vi "PH_VacuumControl.prepare historical Multi Data.vi"(5 "Continue Fit":dbl, 6 "Pressure Data 1 [mbar]":dbl[](array[numeric]), 7 "Start Fit":dbl, 8 "Limit":dbl, 9 "Timebase [s]":i32[](array[numeric]), 10 "Pressure Data 2 [mbar]":dbl[](array[numeric])) -> (1 "Trend":cluster{i32[], "Data":dbl[]}[](graph), 2 "Time to reach Limit":dbl)   [LabVIEW 2014, in "PH_VacuumControl.lvlib"]
doc: "Within this VI the data are prepared for presentation at the GUI and a trend calculation is tried."
uses:
  PH_VacuumControl.lvlib
  <vilib>/Analysis/NI_AALPro.lvlib
panel:
  in  "parameter bounds":T1={"amp min"=-inf, "amp max"=inf, "damping min"=-inf, "damping max"=inf, "offset min"=0.0, "offset max"=0.0}
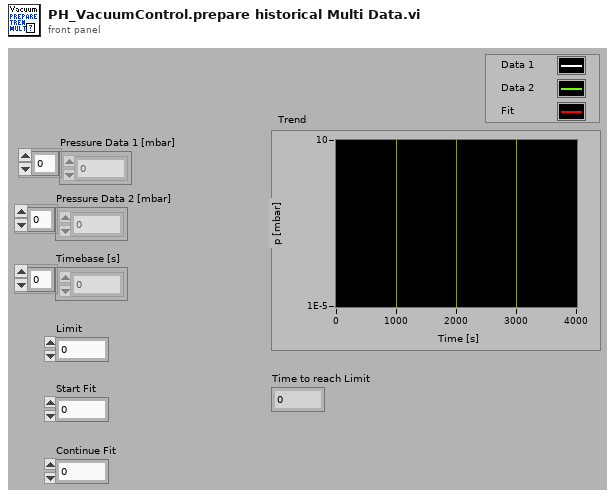
[diagram p1: front panel]
types:
  T1 = cluster{"amp min":dbl, "amp max":dbl, "damping min":dbl, "damping max":dbl, "offset min":dbl, "offset max":dbl}
  T2 = cluster{"Timebase [s]":i32[], "Pressure Data 1 [mbar]":dbl[]}
  T3 = cluster{"Timebase [s]":i32[], "Pressure Data 2 [mbar]":dbl[]}
  T4 = cluster{"Timebase [s]":i32[], "Best Exponential Fit":dbl[]}[]
  T5 = cluster{"Timebase [s]":i32[], "Pressure Data 2 [mbar]":dbl[]}[]
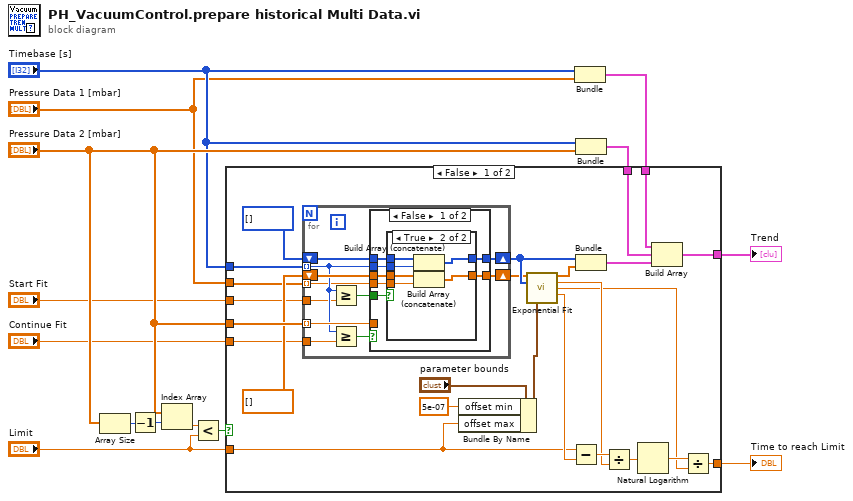
[diagram p0: block diagram]
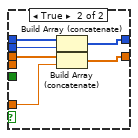
[diagram p3: hidden frame]
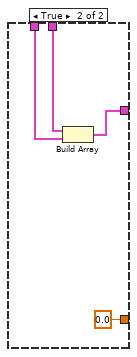
[diagram p4: hidden frame]
diagram:
  n1 = Array Size(array="Pressure Data 2 [mbar]") -> (size(s)=w13:i32)
  n2 = Decrement(x=w13) -> (x-1=w11:i32)
  n3 = Index Array(array="Pressure Data 2 [mbar]", index=w11) -> (element=w10:dbl)
  n4 = Less?(x=w10, y="Limit") -> (x < y?=w8:bool)
  n5 = Bundle("Timebase [s]"="Timebase [s]", "Pressure Data 1 [mbar]"="Pressure Data 1 [mbar]") -> (w4:T2)  [unwired: 1 in]
  n6 = Bundle("Timebase [s]"="Timebase [s]", "Pressure Data 2 [mbar]"="Pressure Data 2 [mbar]") -> (w6:T3)  [unwired: 1 in]
  n7 = case shown="False" w8 {
    tunnel: w6 -> [w18 w75]
    tunnel: [w32 0.0] -> w14
    tunnel: "Timebase [s]" -> [w28 _]
    tunnel: "Pressure Data 2 [mbar]" -> [w27 _]
    tunnel: "Continue Fit" -> [w22 _]
    tunnel: "Limit" -> [w21 _]
    tunnel: [w19 w74] -> w7
    tunnel: w4 -> [w17 w72]
    tunnel: "Pressure Data 1 [mbar]" -> [w15 _]
    tunnel: "Start Fit" -> [w16 _]
    frame False {
      n8 = for {
        tunnel: w28 -> [w43] mode=indexing
        tunnel: w27 -> [w44] mode=indexing
        tunnel: w22 -> [w50]
        shift-right: [w48] -> w26
        shift-left: i32[] [] -> [w47]
        shift-right: [w46] -> w25
        shift-left: dbl[] [] -> [w45]
        tunnel: w16 -> [w42]
        tunnel: w15 -> [w40] mode=indexing
        n9 = Greater Or Equal?(x=w43, y=w42) -> (x >= y?=w41:bool)
        n10 = Greater Or Equal?(x=w43, y=w50) -> (x >= y?=w49:bool)
        n11 = case shown="False" w49 {
          tunnel: w43 -> [w57 w71]
          tunnel: [w55 w70] -> w48
          tunnel: w47 -> [w56 w69]
          tunnel: [w53 w68] -> w46
          tunnel: w45 -> [w54 w67]
          tunnel: w44 -> [_ w66]
          tunnel: w41 -> [w52 _]
          tunnel: w40 -> [w51 _]
          frame False {
            n12 = case shown="True" w52 {
              tunnel: w57 -> [_ w65]
              tunnel: w56 -> [w59 w64]
              tunnel: [w59 w63] -> w55
              tunnel: w54 -> [w58 w62]
              tunnel: [w58 w61] -> w53
              tunnel: w51 -> [_ w60]
              frame False {
              }
              frame True {
                n13 = Build Array (concatenate)(w64, w65) -> (w63:i32[])
                n14 = Build Array (concatenate)(w62, w60) -> (w61:dbl[])
              }
            }
          }
          frame True {
            n15 = Build Array (concatenate)(w69, w71) -> (w70:i32[])
            n16 = Build Array (concatenate)(w67, w66) -> (w68:dbl[])
          }
        }
      }
      n17 = Bundle By Name(cluster="parameter bounds", "offset min"=5e-07, "offset max"=w21) -> (w30:T1)
      n18 = call <vilib>:"Exponential Fit.vi"("Y"=w25, "X"=w26, "parameter bounds"=w30) -> ("Best Exponential Fit"=w39:dbl[], "amplitude"=w36:dbl, "damping"=w33:dbl, "offset"=w38:dbl)  [unwired: 7 in, 2 out]
      n19 = Subtract(x=w21, y=w38) -> (x-y=w37:dbl)
      n20 = Bundle(w26, "Best Exponential Fit"=w39) -> (w20:cluster{i32[], "Best Exponential Fit":dbl[]})  [unwired: 1 in]
      n21 = Divide(x=w37, y=w36) -> (x/y=w35:dbl)
      n22 = Natural Logarithm(1:w35) -> (0:w34:dbl)
      n23 = Build Array(w17, w18, w20) -> (w19:T4)
      n24 = Divide(x=w34, y=w33) -> (x/y=w32:dbl)
    }
    frame True {
      n25 = Build Array(w72, w75) -> (w74:T5)
    }
  }
  "Trend" <- w7
  "Time to reach Limit" <- w14
